vi "Adress counter.vi"(8 "input valid":bool=TRUE, 11 "Reset":bool) -> (0 "output valid":bool, 2 "Address":u32)   [LabVIEW 2013]
uses:
  Program/National Instruments/LabVIEW 2013/instr.lib/_niInstr/Basic Elements/v1/FPGA/Private/Count Up U32.vi
  Program/National Instruments/LabVIEW 2013/instr.lib/_niInstr/Basic Elements/v1/FPGA/niInstr Basic Elements v1 FPGA.lvlib
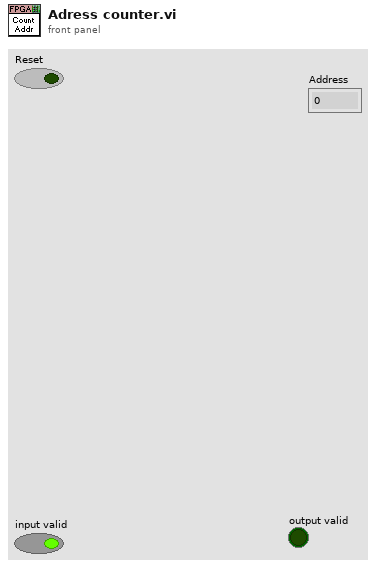
[diagram p1: front panel]
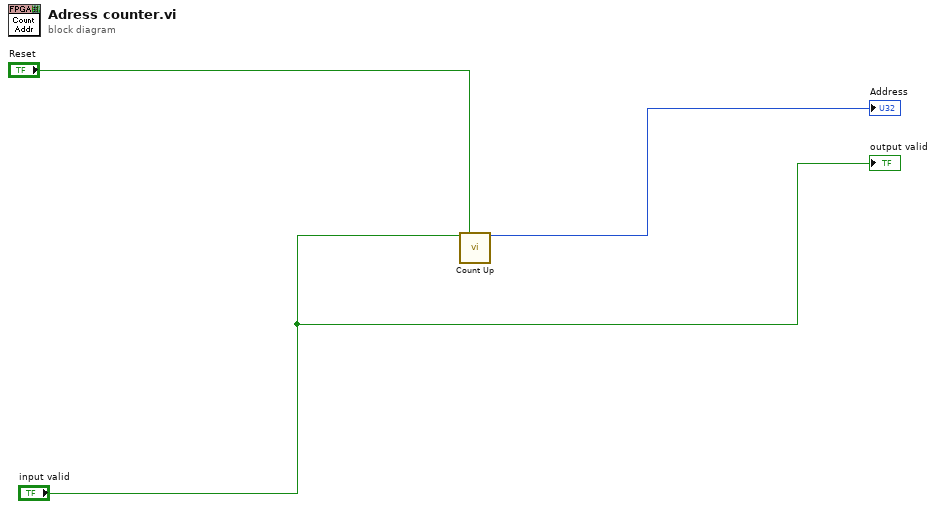
[diagram p0: block diagram]
diagram:
  n1 = call-poly "Count Up.vi"("increment"="input valid", "reset"="Reset") -> ("count out"=→"Address":u32)  [unwired: 13 in]
  "output valid" <- "input valid"
